vi "Gen_FetchData_QX.vi"(8 "Error in":errorcluster, 10 "Cards":T2[](array[typedef]), 11 "QXDAQ reference":refnum<k24>) -> (0 "Fehler (Ausgang)":errorcluster, 2 "Data Out":T1[](array[typedef]))   [LabVIEW 2016]
uses:
  Hardware Drivers/QX/DAQ_ReadBlock.ctl
  DAQ-Config/Controls/PSCHN_Channel Para.ctl
  DAQ-Config/Controls/PSCHN_Card Para.ctl
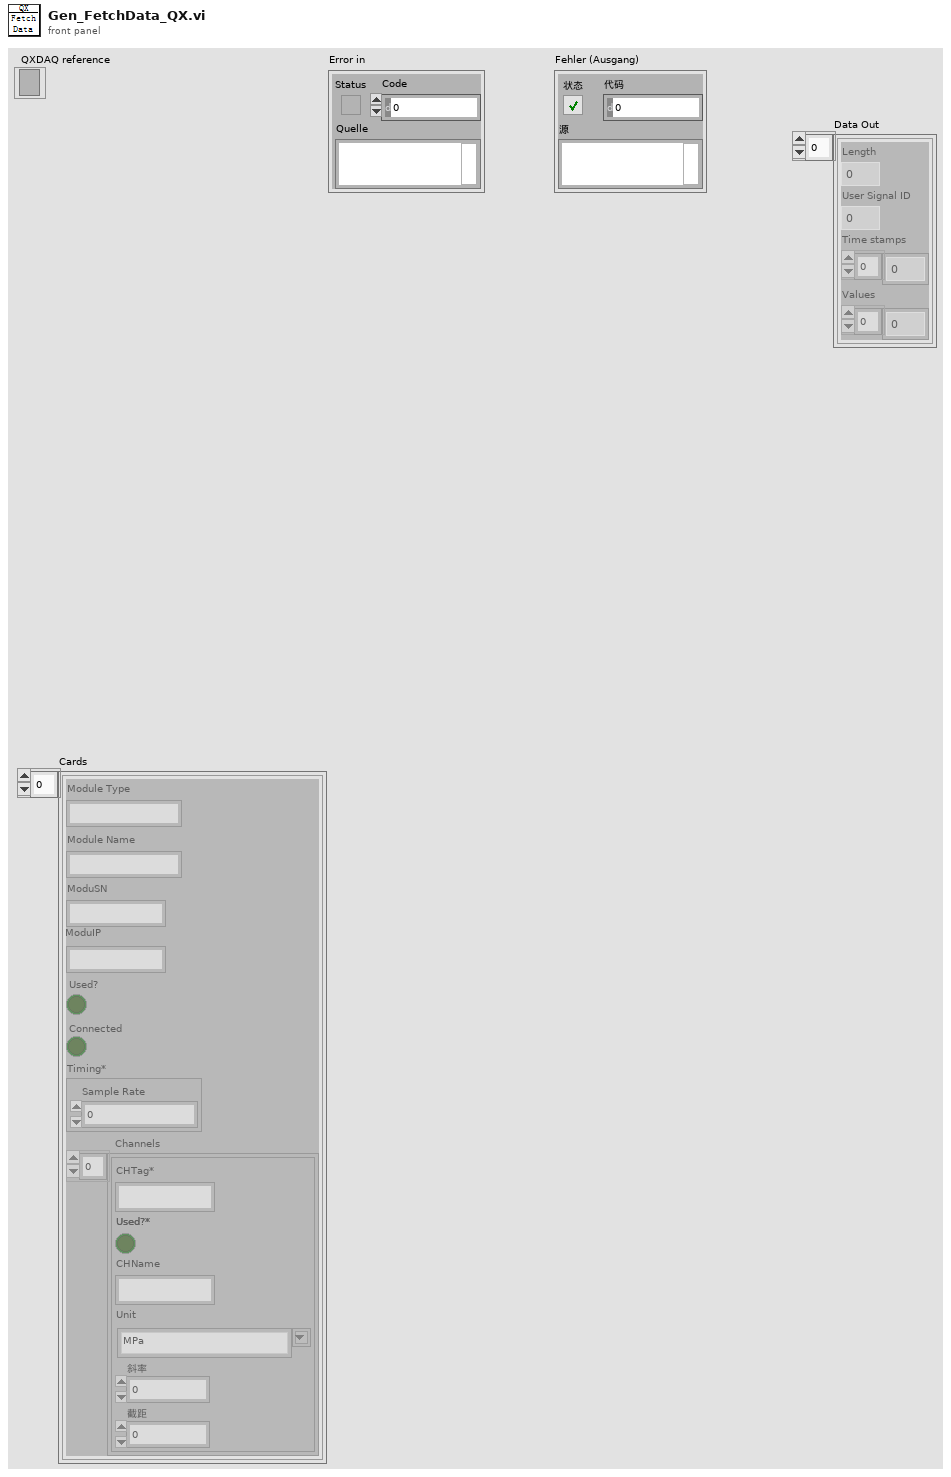
[diagram p1: front panel]
types:
  T1 = typedef "DAQ_ReadBlock.ctl" = cluster{"Length":i32, "User Signal ID":i32, "Time stamps":dbl[], "Values":dbl[]}
  T2 = typedef "PSCHN_Card Para.ctl" = cluster{"Module Type":string, "Module Name":string, "ModuSN":string, "ModuIP":string, "Used?":bool, "Connected":bool, "Timing*":cluster{"Sample Rate":dbl}, "Channels":T3[]}
  T3 = typedef "PSCHN_Channel Para.ctl" = cluster{"CHTag*":string, "Used?*":bool, "CHName":string, "Unit":string, "斜率":dbl, "截距":dbl}
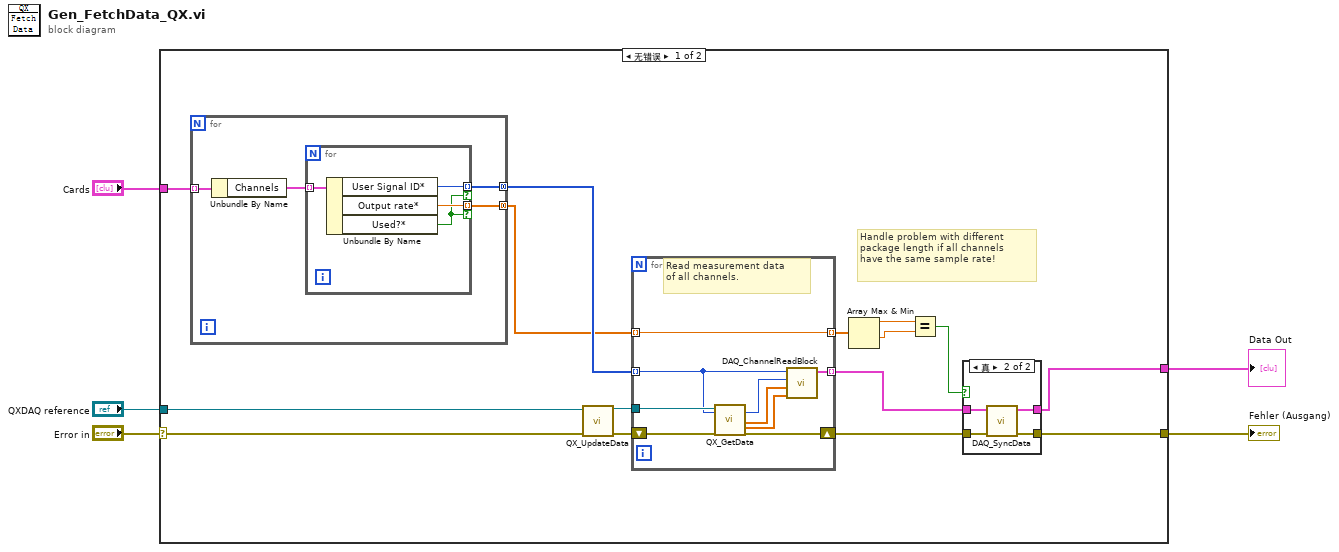
[diagram p0: block diagram]
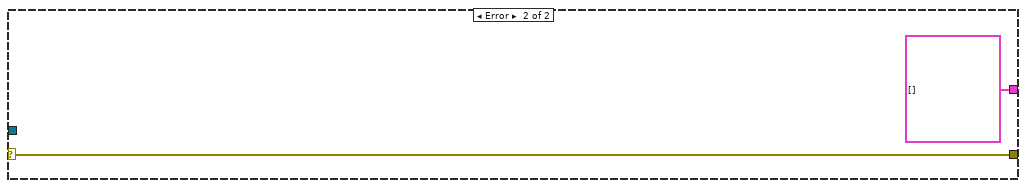
[diagram p3: hidden frame]
diagram:
  n1 = case shown="无错误" "Error in" {
    selector: "Error in" -> [w10 w45]
    tunnel: "Cards" -> [w13 _]
    tunnel: [w9 w45] -> w3
    tunnel: "QXDAQ reference" -> [w7 _]
    tunnel: [w6 T1[] [] ("Data Out")] -> w1
    frame No Error {
      # "Handle problem with different\npackage length if all channels\nhave the same sample rate!"
      n2 = for {
        tunnel: w13 -> [w24] mode=indexing
        tunnel: [w22] -> w12 mode=concatenating
        tunnel: [w21] -> w11 mode=concatenating
        n3 = Unbundle By Name(w24) -> ("Channels"=w23:T3[])
        n4 = for {
          tunnel: w23 -> [w28] mode=indexing
          tunnel: [w27] -> w22 mode=indexing if=w25
          tunnel: [w26] -> w21 mode=indexing if=w25
          n5 = Unbundle By Name(w28) -> ("User Signal ID*"=w27:i32, "Output rate*"=w26:dbl, "Used?*"=w25:bool)
        }
      }
      n6 = call <userlib>:"QX_UpdateData.vi"("Error in"=w10, "QXDAQ reference"=w7) -> ("Error out"=w20:errorcluster, "QXDAQ reference"=w19:refnum<k24>)  [unwired: 8 in]
      n7 = for {
        tunnel: w19 -> [w42]
        shift-right: [w41] -> w17
        shift-left: w20 -> [w43]
        tunnel: [w38] -> w18 mode=indexing
        tunnel: [w35] -> w8 mode=indexing
        tunnel: w12 -> [w36] mode=indexing
        tunnel: w11 -> [w35] mode=indexing
        # "Read measurement data\nof all channels."
        n8 = call <userlib>:"QX_GetData.vi"("QXDAQ reference"=w42, "UserSignalID"=w36, "Error in"=w43) -> ("Count"=w40:i32, "Time stamps"=w39:dbl[], "Values"=w37:dbl[], "Error out"=w41:errorcluster)  [unwired: 11 in, 2 out]
        n9 = call "DAQ_ChannelReadBlock.vi"("User Signal ID"=w36, "Count"=w40, "Time stamps"=w39, "Values"=w37) -> ("Read block"=w38:T1)  [unwired: 6 in]
      }
      n10 = Array Max & Min(array=w8) -> (max value=w15:dbl, min value=w16:dbl)  [unwired: 2 out]
      n11 = Equal?(x=w15, y=w16) -> (x = y?=w14:bool)
      n12 = case shown="真" w14 {
        tunnel: w18 -> [w30 w34]
        tunnel: w17 -> [w29 w33]
        tunnel: [w29 w32] -> w9
        tunnel: [w30 w31] -> w6
        frame False {
        }
        frame True {
          n13 = call "DAQ_SyncData.vi"("Fehler (Eingang)"=w33, "Data In"=w34) -> ("Fehler (Ausgang)"=w32:errorcluster, "Data Out"=w31:T1[])  [unwired: 6 in, 2 out]
        }
      }
    }
    frame Error {
    }
  }
  "Fehler (Ausgang)" <- w3
  "Data Out" <- w1
